vi "RTS Index Sorted Filenames.vi"(6 "Base File Name":string, 8 "Error In":errorcluster, 9 "Sorted Filename index":i32[](array[numeric]), 10 "filenames":string[](array[string]), 11 "stripped path":path) -> (0 "Error Out":errorcluster, 2 "Full Data List":path[](array[path]), 3 "Organized File Open List":path[](array[path]))   [LabVIEW 2016]
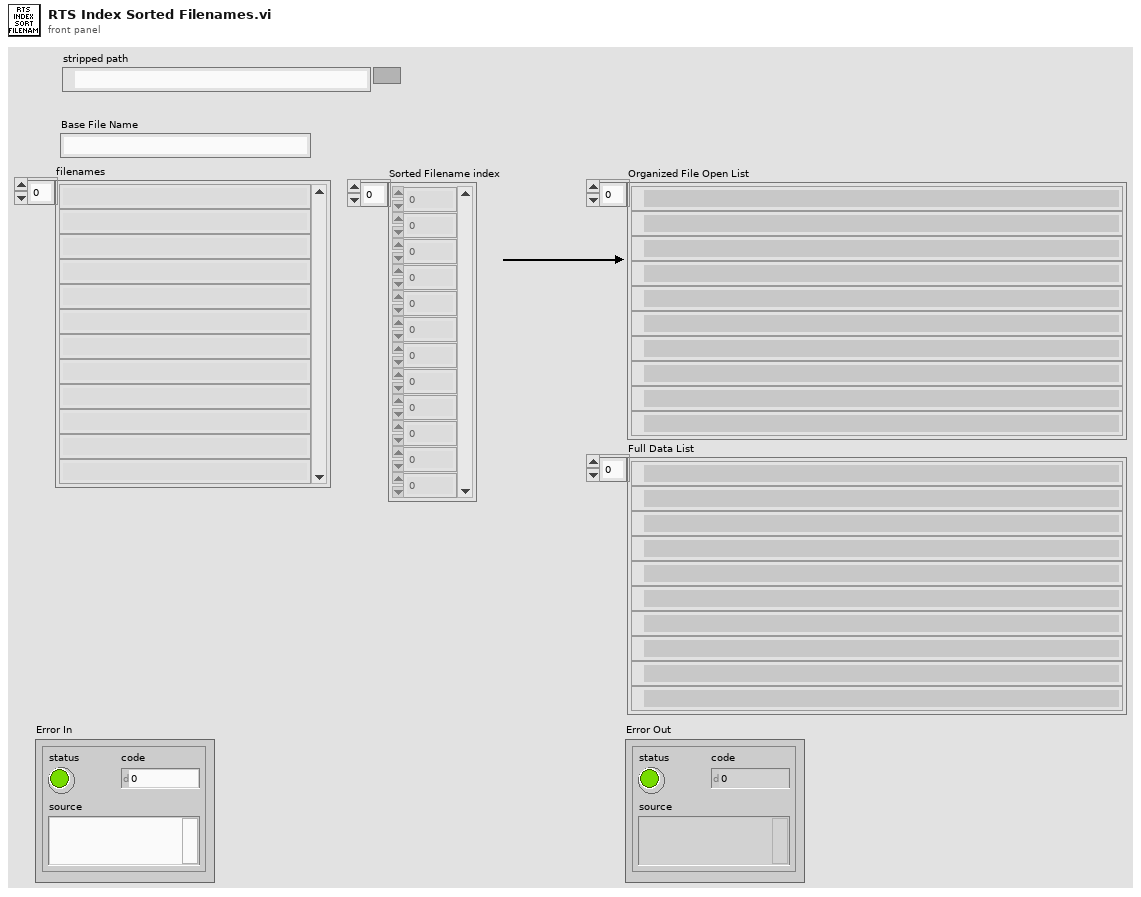
[diagram p1: front panel]
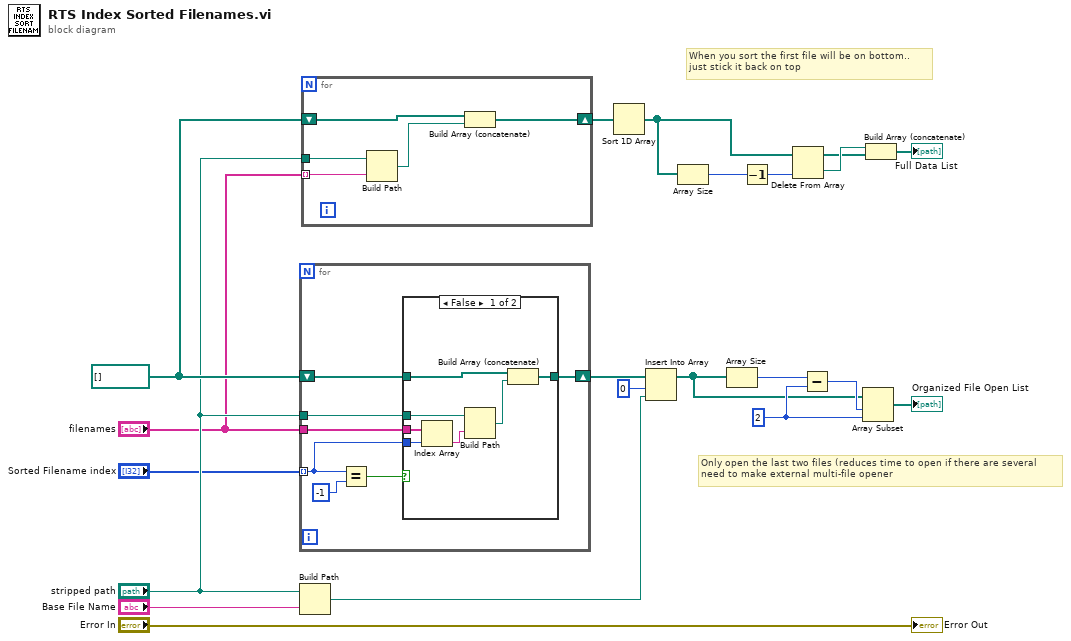
[diagram p0: block diagram]
diagram:
  w16 = 2 ("length")
  w11 = path[] []
  # "When you sort the first file will be on bottom..\njust stick it back on top"
  # "Only open the last two files (reduces time to open if there are several\nneed to make external multi-file opener"
  n1 = for {
    tunnel: "Sorted Filename index" -> [w28] mode=indexing
    tunnel: "filenames" -> [w25]
    shift-right: [w23] -> w13
    shift-left: w11 -> [w24]
    tunnel: "stripped path" -> [w22]
    n2 = Equal?(x=w28, y=-1) -> (x = y?=w26:bool)
    n3 = case shown="False" w26 {
      tunnel: w28 -> [w34 _]
      tunnel: w25 -> [w35 _]
      tunnel: w24 -> [w33 w36]
      tunnel: [w32 w36] -> w23
      tunnel: w22 -> [w31 _]
      frame False {
        n4 = Index Array(array=w35, index=w34) -> (element=w30:string)
        n5 = Build Path(base path=w31, name or relative path=w30) -> (appended path=w29:path)
        n6 = Build Array (concatenate)(w33, w29) -> (w32:path[])
      }
      frame True {
      }
    }
  }
  n7 = Build Path(base path="stripped path", name or relative path="Base File Name") -> (appended path=w20:path)
  n8 = for {
    tunnel: "filenames" -> [w37] mode=indexing
    shift-right: [w40] -> w7
    shift-left: w11 -> [w41]
    tunnel: "stripped path" -> [w39]
    n9 = Build Path(base path=w39, name or relative path=w37) -> (appended path=w38:path)
    n10 = Build Array (concatenate)(w41, w38) -> (w40:path[])
  }
  n11 = Sort 1D Array(array=w7) -> (sorted array=w6:path[])
  n12 = Insert Into Array(array=w13, index=0, new element=w20) -> (w12:path[])
  n13 = Array Size(array=w6) -> (size(s)=w5:i32)
  n14 = Array Size(array=w12) -> (size(s)=w15:i32)
  n15 = Decrement(x=w5) -> (x-1=w4:i32)
  n16 = Delete From Array(array=w6, index=w4) -> (deleted portion=w3:path, array with subset deleted=w2:path[])  [unwired: 1 in]
  n17 = Subtract(x=w15, y=w16) -> (x-y=w17:i32)
  n18 = Array Subset(array=w12, index=w17, length=w16) -> (→"Organized File Open List":path[])
  n19 = Build Array (concatenate)(w3, w2) -> (→"Full Data List":path[])
  "Error Out" <- "Error In"
